vi "SubVI_CinematicaDireta.vi"() -> ()   [LabVIEW 2017]
uses:
  <vilib>/Analysis/coordinate.llb/Angle Units.ctl
  <vilib>/Analysis/coordinate.llb/Wrap Angle (array).vi
  <vilib>/robotics/Kinematics/Robot/Forward Kinematics (Point).vi
  <vilib>/picture/3D Picture Control/Object/Add Object (reference).vi
  <vilib>/robotics/Kinematics/Plotting/NI_Robotics_3DKinematics.lvlib
  <vilib>/picture/3D Picture Control/NI_3D Picture Control.lvlib
  <vilib>/robotics/Kinematics/NI_Kinematics.lvlib
  <vilib>/Analysis/NI_AAL_Angle.lvlib
panel:
  out "angles":cluster{"roll":dbl, "pitch":dbl, "yaw":dbl}
  out "translation vector":dbl[](array[numeric])
  out "error out":errorcluster
  out "3D Picture Control":refnum<vi>(3d-picture)
  in  "joint positions":dbl[](array[numeric])
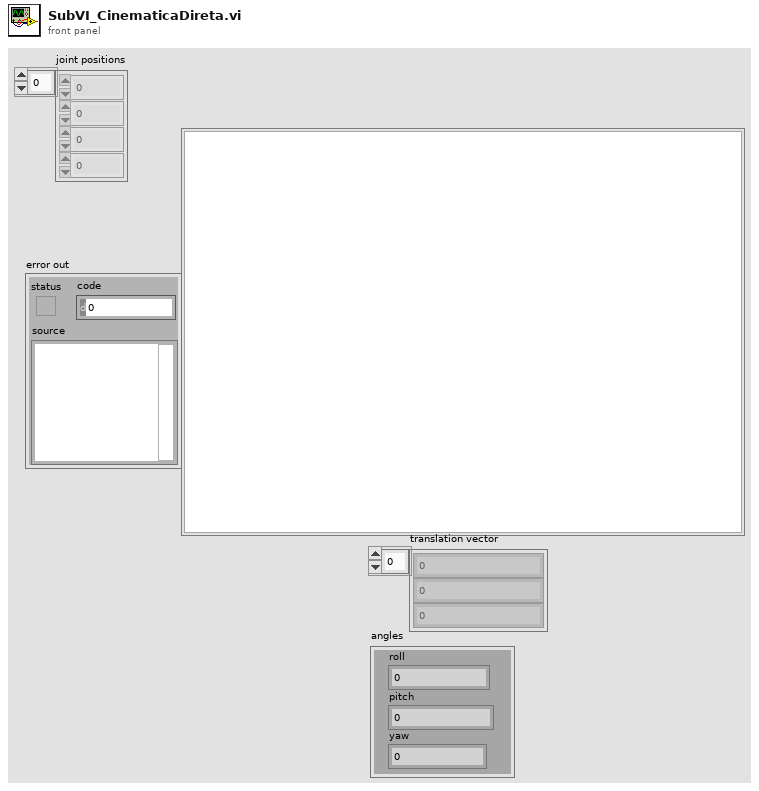
[diagram p1: front panel]
types:
  T1 = typedef "NI_AAL_Angle.lvlib/Angle Units.ctl" = i32
  T2 = typedef "NI_Matrix.lvlib/RealMatrix.ctl" = dbl[][]
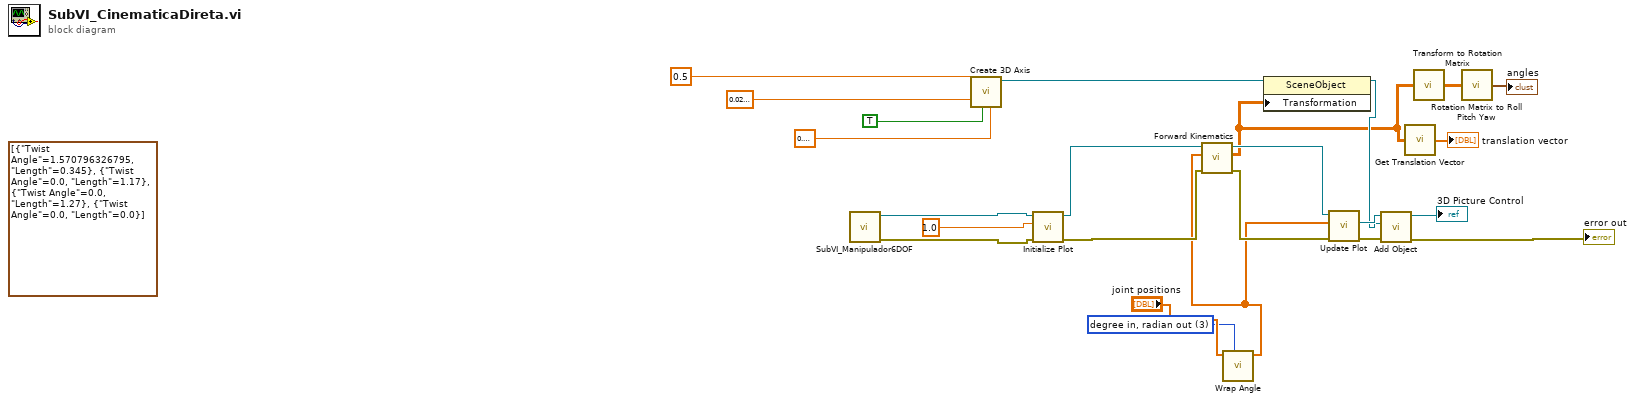
[diagram p0: block diagram]
diagram:
  w3 = T1 3 items=["radian in, radian out", "radian in, degree out", "degree in, degree out", "degree in, radian out"] ("angle units")
  (unwired) cluster{"Twist Angle":dbl, "Length":dbl}[] [{"Twist Angle"=1.570796326795, "Length"=0.345}, {"Twist Angle"=0.0, "Length"=1.17}, {"Twist Angle"=0.0, "Length"=1.27}, {"Twist Angle"=0.0, "Length"=0.0}]
  n1 = call "SubVI_Manipulador6DOF.vi"() -> ("error out"=w1:errorcluster, "NI_Robotics_Serial Robot Arm out"=w2:refnum<class "NI_Robotics_Serial Robot Arm.lvclass">)  [unwired: 10 in]
  n2 = call <vilib>:"Create 3D Axis.vi"("Character Size"=sgl 0.2, "Axis label?"=TRUE, "Radius"=sgl 0.03, "Length"=sgl 0.5) -> ("New Object Refnum"=w17:refnum<vi>)  [unwired: 6 in, 1 out]
  n3 = call <vilib>:"Initialize Plot.vi"("error in (no error)"=w1, "scale (1)"=1.0, "serial arm in"=w2) -> ("error out"=w18:errorcluster, "serial arm out"=w19:refnum<class "NI_Robotics_Serial Robot Arm.lvclass">)  [unwired: 7 in]
  n4 = call-poly <vilib>:"Wrap Angle.vi"("angle units"=w3, "Angle In"="joint positions") -> ("Angle Out"=w4:dbl[])  [unwired: 8 in, 1 out]
  n5 = call-poly <vilib>:"Forward Kinematics.vi"("error in (no error)"=w18, "joint positions"=w4, "serial arm in"=w19) -> ("error out"=w15:errorcluster, "end effector transform"=w8:T2, "serial arm out"=w14:refnum<class "NI_Robotics_Serial Robot Arm.lvclass">)  [unwired: 6 in]
  n6 = property class="SceneObject"(reference=w17, "Transformation"=w8) -> (reference out=w11:refnum<vi>)  [unwired: 1 in, 1 out]
  n7 = call <vilib>:"Update Plot.vi"("error in (no error)"=w15, "joint positions"=w4, "serial arm in"=w14) -> ("error out"=w13:errorcluster, "serial arm scene"=w12:refnum<vi>)  [unwired: 6 in, 1 out]
  n8 = call-poly <vilib>:"Add Object.vi"("error in (no error)"=w13, "New Object In"=w11, "Scene Object In"=w12) -> ("error out"=→"error out":errorcluster, "Scene Object Out"=→"3D Picture Control":refnum<vi>)  [unwired: 6 in, 1 out]
  n9 = call <vilib>:"Get Translation Vector.vi"("transform"=w8) -> ("translation vector"=→"translation vector":dbl[])
  n10 = call <vilib>:"Transform to Rotation Matrix.vi"("transform"=w8) -> ("rotation matrix"=w7:T2)
  n11 = call <vilib>:"Rotation Matrix to Roll Pitch Yaw.vi"("rotation matrix"=w7) -> ("angles"=→"angles":cluster{"roll":dbl, "pitch":dbl, "yaw":dbl})
